vi "LEDExecute.vi"   [LabVIEW 2023]
uses:
  <vilib>/Rock Robotics/WPI/ThirdParty/PhotonVisionLib/PhotonVisionLib.lvlib
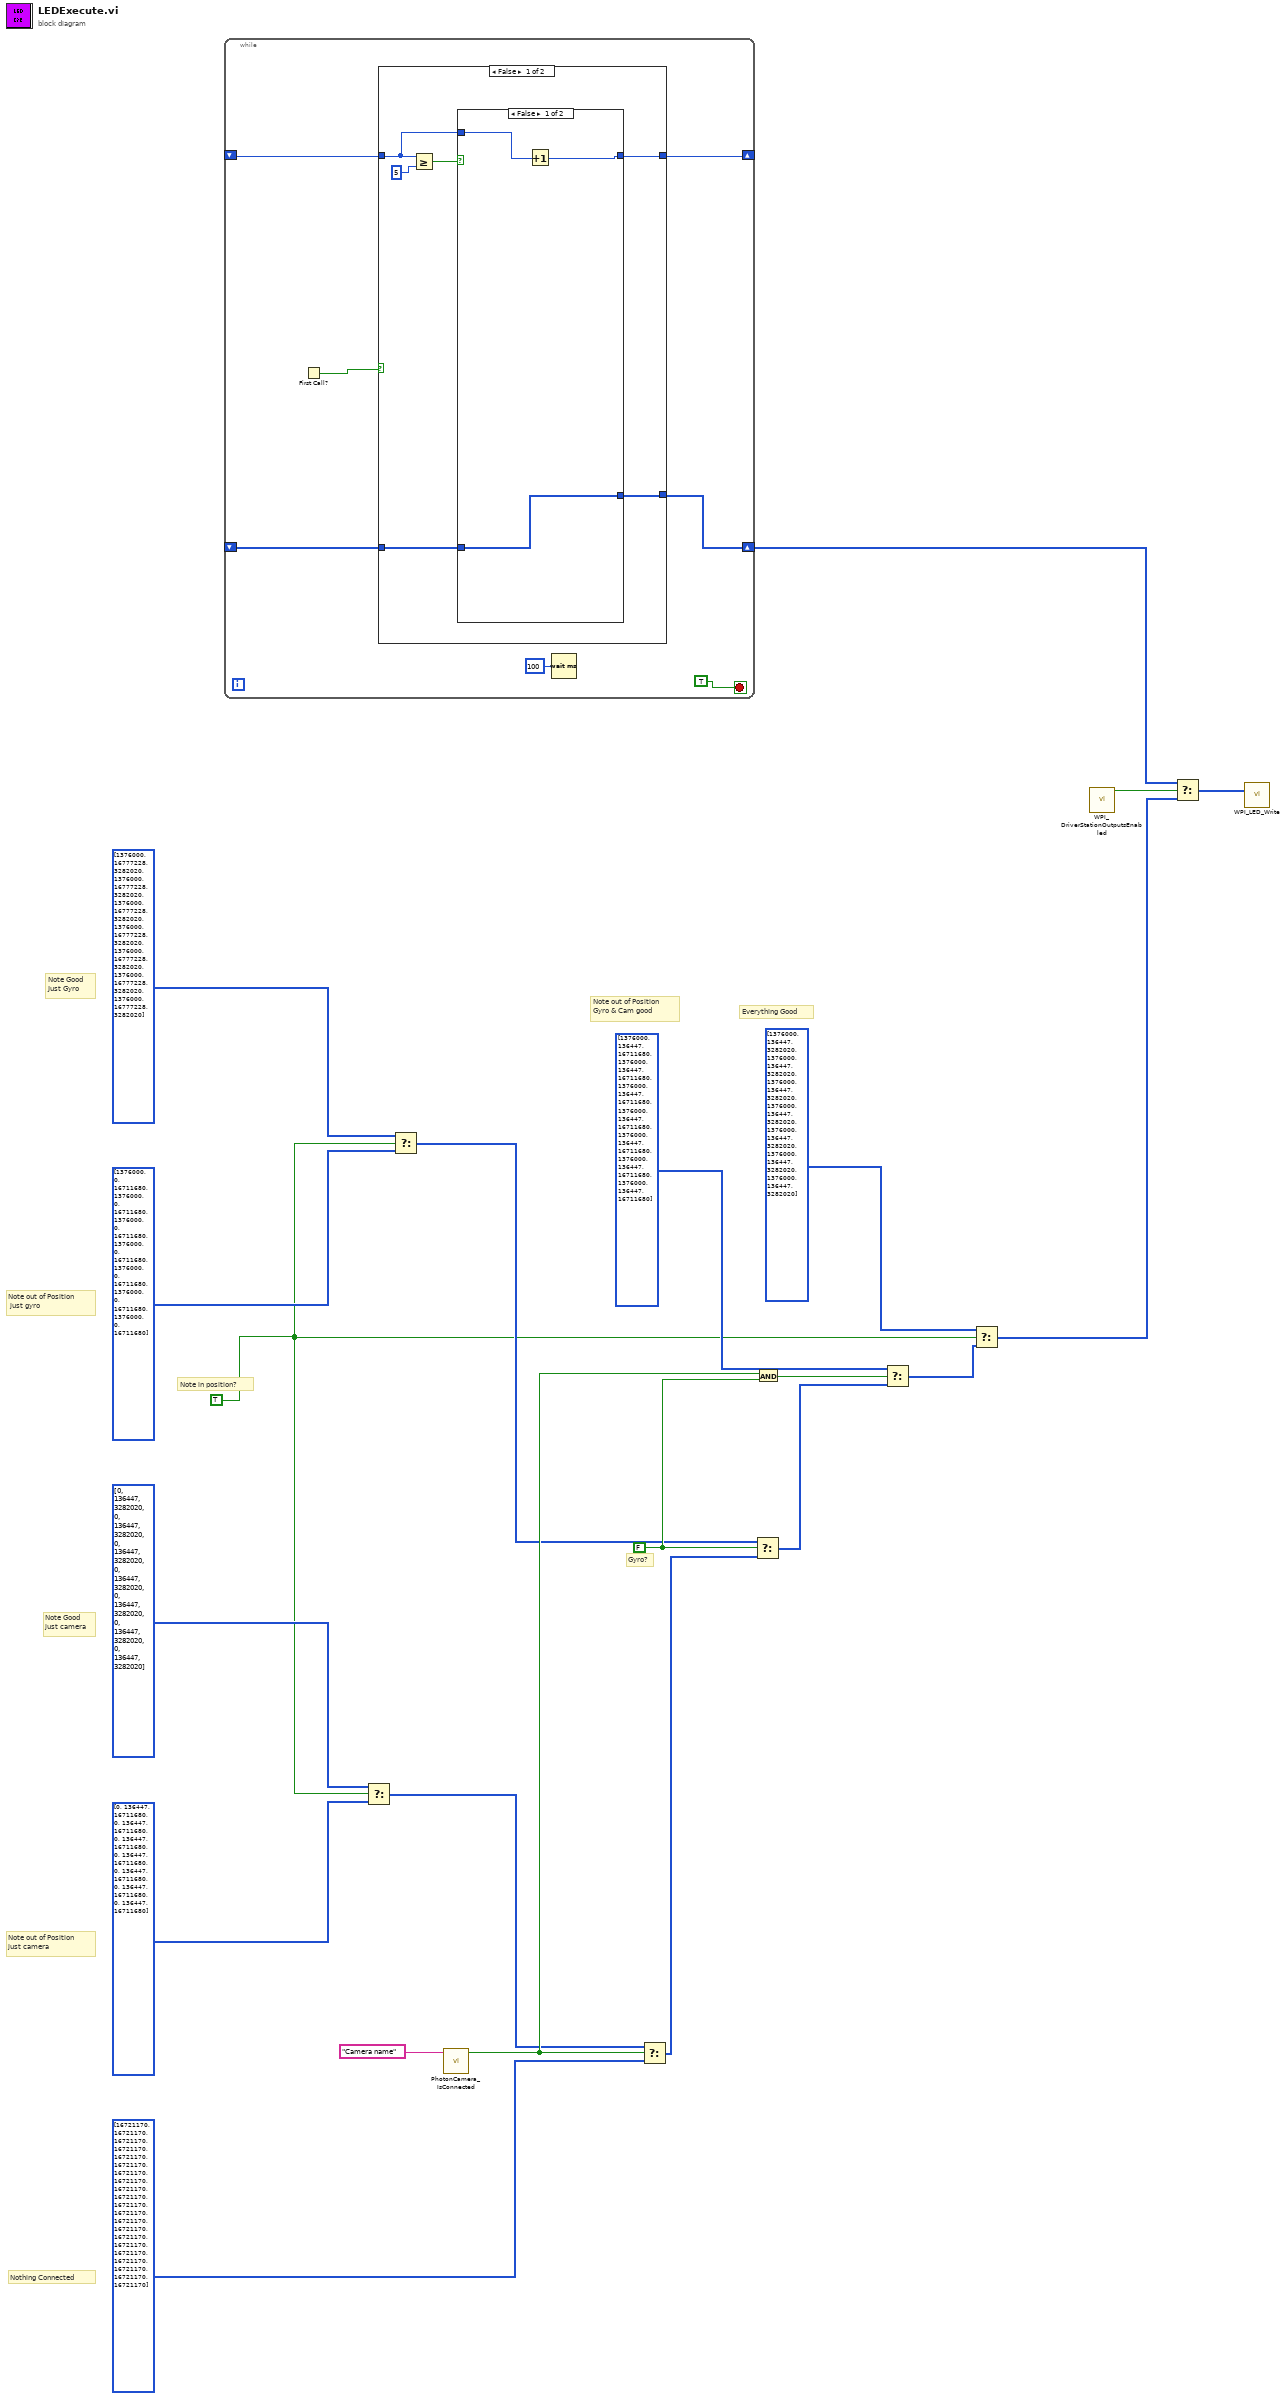
[diagram p0: block diagram]
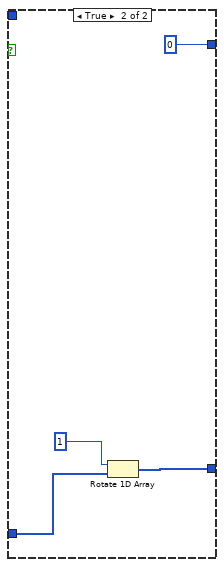
[diagram p2: hidden frame]
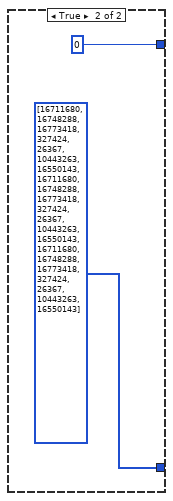
[diagram p3: hidden frame]
diagram:
  w1 = TRUE
  w17 = FALSE
  # "Note Good\njust camera"
  # "Note Good\nJust Gyro"
  # "Note in position?"
  # "Note out of Position\n just gyro"
  # "Note out of Position\njust camera"
  # "Everything Good"
  # "Note out of Position\nGyro & Cam good"
  # "Gyro?"
  # "Nothing Connected"
  n1 = while {
    shift-right: [w26] -> w12
    shift-left: _ -> [w23]
    shift-right: [w25] -> _
    shift-left: _ -> [w24]
    stop <- TRUE stop-if-true
    n2 = First Call?() -> (First Call?: T/F=w27:bool)
    n3 = case shown="False" w27 {
      tunnel: [w31 u32[] [16711680, 16748288, 16773418, 327424, 26367, 10443263, 16550143, 16711680, 16748288, 16773418, 327424, 26367, 10443263, 16550143, 16711680, 16748288, 16773418, 327424, 26367, 10443263, 16550143] ("Color Array")] -> w26
      tunnel: [w30 0] -> w25
      tunnel: w24 -> [w29 _]
      tunnel: w23 -> [w32 _]
      frame False {
        n4 = Greater Or Equal?(x=w29, y=5) -> (x >= y?=w33:bool)
        n5 = case shown="False" w33 {
          tunnel: w32 -> [w35 w40]
          tunnel: [w35 w39] -> w31
          tunnel: [w37 0] -> w30
          tunnel: w29 -> [w36 _]
          frame False {
            n6 = Increment(x=w36) -> (x+1=w37:i32)
          }
          frame True {
            n7 = Rotate 1D Array(1:w40, 2:1 ("n")) -> (0:w39:u32[])
          }
        }
      }
      frame True {
      }
    }
    n8 = Wait (ms)(milliseconds to wait=u32 100) -> ()  [unwired: 1 out]
  }
  n9 = Select(t=u32[] [0, 136447, 3282020, 0, 136447, 3282020, 0, 136447, 3282020, 0, 136447, 3282020, 0, 136447, 3282020, 0, 136447, 3282020, 0, 136447, 3282020] ("Color Array"), s=w1, f=u32[] [0, 136447, 16711680, 0, 136447, 16711680, 0, 136447, 16711680, 0, 136447, 16711680, 0, 136447, 16711680, 0, 136447, 16711680, 0, 136447, 16711680] ("Color Array")) -> (s? t:f=w8:u32[])
  n10 = Select(t=u32[] [1376000, 16777228, 3282020, 1376000, 16777228, 3282020, 1376000, 16777228, 3282020, 1376000, 16777228, 3282020, 1376000, 16777228, 3282020, 1376000, 16777228, 3282020, 1376000, 16777228, 3282020] ("Color Array"), s=w1, f=u32[] [1376000, 0, 16711680, 1376000, 0, 16711680, 1376000, 0, 16711680, 1376000, 0, 16711680, 1376000, 0, 16711680, 1376000, 0, 16711680, 1376000, 0, 16711680] ("Color Array")) -> (s? t:f=w10:u32[])
  n11 = call <vilib>:"PhotonCamera_IsConnected.vi"("CameraName"="Camera name") -> ("IsConnected"=w15:bool)  [unwired: 9 in, 1 out]
  n12 = Select(t=w8, s=w15, f=u32[] [16721170, 16721170, 16721170, 16721170, 16721170, 16721170, 16721170, 16721170, 16721170, 16721170, 16721170, 16721170, 16721170, 16721170, 16721170, 16721170, 16721170, 16721170, 16721170, 16721170, 16721170] ("Color Array")) -> (s? t:f=w21:u32[])
  n13 = Select(t=w10, s=w17, f=w21) -> (s? t:f=w19:u32[])
  n14 = And(x=w15, y=w17) -> (x .and. y?=w18:bool)
  n15 = Select(t=u32[] [1376000, 136447, 16711680, 1376000, 136447, 16711680, 1376000, 136447, 16711680, 1376000, 136447, 16711680, 1376000, 136447, 16711680, 1376000, 136447, 16711680, 1376000, 136447, 16711680] ("Color Array"), s=w18, f=w19) -> (s? t:f=w5:u32[])
  n16 = Select(t=u32[] [1376000, 136447, 3282020, 1376000, 136447, 3282020, 1376000, 136447, 3282020, 1376000, 136447, 3282020, 1376000, 136447, 3282020, 1376000, 136447, 3282020, 1376000, 136447, 3282020] ("Color Array"), s=w1, f=w5) -> (s? t:f=w4:u32[])
  n17 = call <vilib>:"WPI_DriverStationOutputsEnabled.vi"() -> ("OutputsEnabled?"=w14:bool)  [unwired: 10 in, 1 out]
  n18 = Select(t=w12, s=w14, f=w4) -> (s? t:f=w13:u32[])
  n19 = call <vilib>:"WPI_LED_Write.vi"("Color Array"=w13) -> ()  [unwired: 10 in, 1 out]
